vi "build.vi"(8 "error in (no error)":errorcluster, 10 "build_spec":T1, 11 "lv-build-default in":refnum<class "lv-builder.lvclass">) -> (0 "error out":errorcluster, 2 "[] generated_files":path[](array[path]), 3 "lv-build-default out":refnum<class "lv-builder.lvclass">)   [LabVIEW 2015, in "lv-builder.lvclass"]
uses:
  lv-builder.lvclass
  lv-build/public/_controls/build_specification.ctl
  lv-build/public/_controls/build_type.ctl
  lv-build/lv-build.lvlib
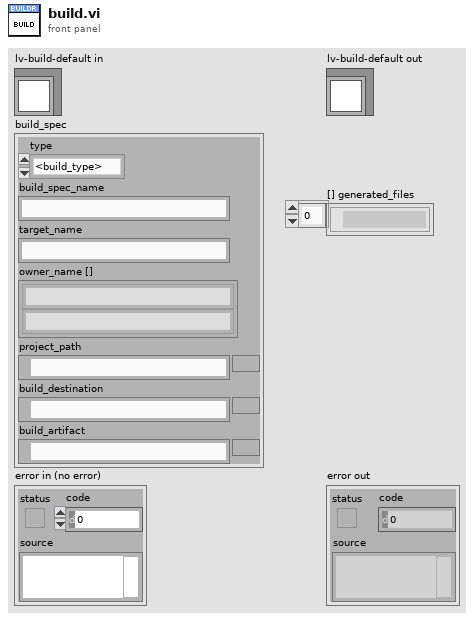
[diagram p1: front panel]
types:
  T1 = typedef "lv-build.lvlib/build_specification.ctl" = cluster{"type":T2, "build_spec_name":string, "target_name":string, "owner_name []":string[], "project_path":path, "build_destination":path, "build_artifact":path}
  T2 = typedef "lv-build.lvlib/build_type.ctl" = enum16{"<build_type>", "application_pc", "application_rt", "installer", "llb", "lvlibp", "zip", "fpga", "<null>"}
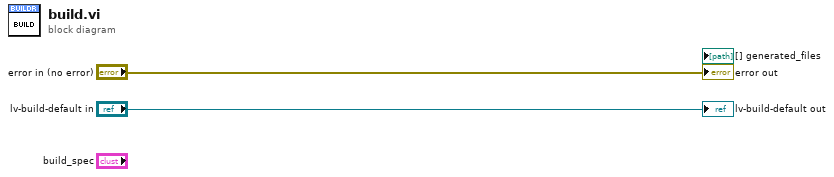
[diagram p0: block diagram]
diagram:
  "error out" <- "error in (no error)"
  "lv-build-default out" <- "lv-build-default in"
